vi "9219_HandleModeChange.vi"(5 "ConfigTD in":T1 {"Conversion Time" items=["High Speed", "Best 60 Hz Rejection", "Best 50 Hz Rejection", "High Resolution"]; "TCoupleType" items=["J", "K", "T", "E", "R", "S", "N", "B"]; "DegreeRange" items=["Raw units", "Degrees Kelvin", "Degrees Celsius", "Degrees Fahrenheit", "Degrees Rankine"]; "RtdType" items=["TCR3851"=1, "TCR3750"=2, "TCR3916"=3, "TCR3920"=4, "TCR3911"=5, "TCR3928"=6, "Custom"=0]}, 7 "New Mode":u8, 9 "Selected Channels":i32[](array[numeric])) -> (6 "ConfigTD out":T1 {"Conversion Time" items=["High Speed", "Best 60 Hz Rejection", "Best 50 Hz Rejection", "High Resolution"]; "TCoupleType" items=["J", "K", "T", "E", "R", "S", "N", "B"]; "DegreeRange" items=["Raw units", "Degrees Kelvin", "Degrees Celsius", "Degrees Fahrenheit", "Degrees Rankine"]; "RtdType" items=["TCR3851"=1, "TCR3750"=2, "TCR3916"=3, "TCR3920"=4, "TCR3911"=5, "TCR3928"=6, "Custom"=0]})   [LabVIEW 2017, in "Modules.lvlib" / "9219.lvclass"]
uses:
  9219.lvclass
  9219 Config.ctl
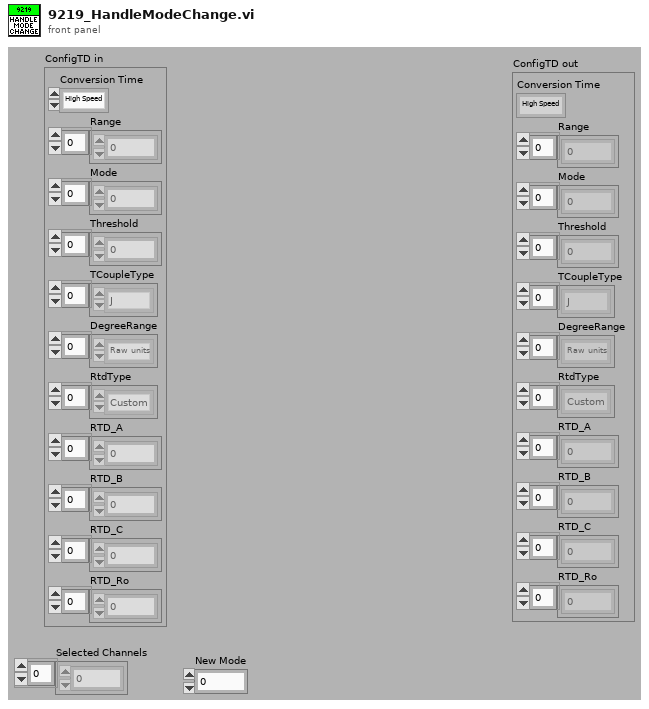
[diagram p1: front panel]
types:
  T1 = typedef "Modules.lvlib/9219.lvclass/9219 Config.ctl" = cluster{"Conversion Time":u16, "Range":u8[], "Mode":u8[], "Threshold":dbl[], "TCoupleType":u8[], "DegreeRange":u8[], "RtdType":u8[], "RTD_A":dbl[], "RTD_B":dbl[], "RTD_C":dbl[], "RTD_Ro":dbl[]}
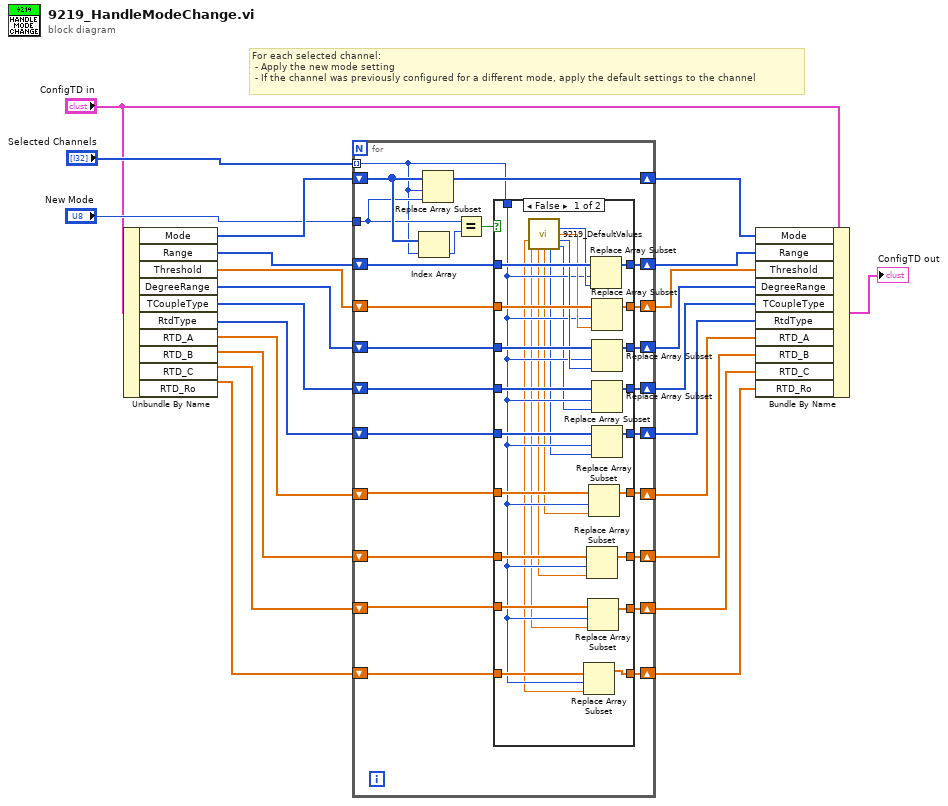
[diagram p0: block diagram]
diagram:
  # "For each selected channel:\n - Apply the new mode setting\n - If the channel was previously configured for a different mode, apply the default settings to the channel"
  n1 = Unbundle By Name("ConfigTD in") -> ("Mode"=w17:u8[], "Range"=w18:u8[], "Threshold"=w19:dbl[], "DegreeRange"=w15:u8[], "TCoupleType"=w14:u8[], "RtdType"=w10:u8[], "RTD_A"=w9:dbl[], "RTD_B"=w8:dbl[], "RTD_C"=w7:dbl[], "RTD_Ro"=w6:dbl[])
  n2 = for {
    tunnel: "New Mode" -> [w45]
    shift-right: [w48] -> w21
    shift-left: w17 -> [w47]
    shift-right: [w42] -> w22
    shift-left: w18 -> [w43]
    shift-right: [w40] -> w23
    shift-left: w19 -> [w41]
    tunnel: "Selected Channels" -> [w39] mode=indexing
    shift-right: [w37] -> w13
    shift-left: w15 -> [w38]
    shift-right: [w35] -> w12
    shift-left: w14 -> [w36]
    shift-right: [w33] -> w5
    shift-left: w10 -> [w34]
    shift-right: [w28] -> w4
    shift-left: w9 -> [w32]
    shift-right: [w27] -> w3
    shift-left: w8 -> [w31]
    shift-right: [w26] -> w2
    shift-left: w7 -> [w30]
    shift-right: [w25] -> w1
    shift-left: w6 -> [w29]
    n3 = Index Array(array=w47, index=w39) -> (element=w46:u8)
    n4 = Replace Array Subset(array=w47, new element=w45, index=w39) -> (w48:u8[])
    n5 = Equal?(x=w45, y=w46) -> (x = y?=w44:bool)
    n6 = case shown="False" w44 {
      tunnel: w43 -> [w76 w85]
      tunnel: [w75 w85] -> w42
      tunnel: w39 -> [w59 _]
      tunnel: w41 -> [w74 w84]
      tunnel: [w73 w84] -> w40
      tunnel: w38 -> [w72 w83]
      tunnel: [w71 w83] -> w37
      tunnel: w36 -> [w70 w82]
      tunnel: [w69 w82] -> w35
      tunnel: w34 -> [w65 w81]
      tunnel: [w64 w81] -> w33
      tunnel: w32 -> [w63 w80]
      tunnel: w31 -> [w62 w79]
      tunnel: w30 -> [w61 w78]
      tunnel: w29 -> [w60 w77]
      tunnel: [w58 w80] -> w28
      tunnel: [w57 w79] -> w27
      tunnel: [w56 w78] -> w26
      tunnel: [w55 w77] -> w25
      frame False {
        n7 = call "9219_DefaultValues.vi"() -> ("Range"=w68:u8, "Threshold"=w67:dbl, "RTD_Ro"=w49:dbl, "Degree Range"=w66:u8, "RTD_C"=w50:dbl, "RTD_B"=w51:dbl, "RTD_A"=w52:dbl, "RTD Types"=w53:u8, "Thermocouple Type"=w54:u8)  [unwired: 5 in, 2 out]
        n8 = Replace Array Subset(array=w60, new element=w49, index=w59) -> (w55:dbl[])
        n9 = Replace Array Subset(array=w62, new element=w51, index=w59) -> (w57:dbl[])
        n10 = Replace Array Subset(array=w61, new element=w50, index=w59) -> (w56:dbl[])
        n11 = Replace Array Subset(array=w63, new element=w52, index=w59) -> (w58:dbl[])
        n12 = Replace Array Subset(array=w76, new element=w68, index=w59) -> (w75:u8[])
        n13 = Replace Array Subset(array=w74, new element=w67, index=w59) -> (w73:dbl[])
        n14 = Replace Array Subset(array=w72, new element=w66, index=w59) -> (w71:u8[])
        n15 = Replace Array Subset(array=w70, new element=w54, index=w59) -> (w69:u8[])
        n16 = Replace Array Subset(array=w65, new element=w53, index=w59) -> (w64:u8[])
      }
      frame True {
        # "mode is unchanged, keep config"
      }
    }
  }
  n17 = Bundle By Name(cluster="ConfigTD in", "Mode"=w21, "Range"=w22, "Threshold"=w23, "DegreeRange"=w13, "TCoupleType"=w12, "RtdType"=w5, "RTD_A"=w4, "RTD_B"=w3, "RTD_C"=w2, "RTD_Ro"=w1) -> (→"ConfigTD out":T1)
